vi "Enqueue Sync Await Release.vi"(8 "error in (no error)":errorcluster, 11 "Instrument Owner in":refnum<class "Instrument Owner.lvclass">) -> (0 "error out":errorcluster, 3 "Instrument Owner out":refnum<class "Instrument Owner.lvclass">)   [LabVIEW 2020, in "Instrument Handler.lvlib" / "Instrument Owner.lvclass"]
doc: "Await a notification on the Enqueue Sync notifier. Wait for Instrument Sequencer to complete the operation."
uses:
  Instrument Owner.lvclass
  Instrument Owner.lvclass/Instrument Owner.ctl
  PPL/HDH.Data.Generic.lvlibp/Synchronization/Notifier/Notifier.lvclass
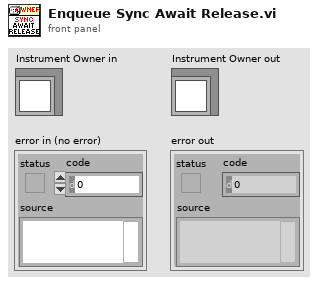
[diagram p1: front panel]
types:
  T1 = typedef "Instrument Handler.lvlib/Ctl_InstrumentSynchronicationCluster.ctl" = cluster{"Launched?":bool, "Driver Path":path, "Alias":string, "Connection Type":T2, "Pre Initialization Data":variant, "Enqueue Sync":refnum<class "Notifier.lvclass">, "Enqueue Lock":T3, "Owner Enqueuer":refnum<class "Message Enqueuer.lvclass">, "Owner":refnum<class "Sequencer Core.lvclass">, "Instrument ID":u32}
  T2 = typedef "HDH.Actor Framework.Core.Instrument Driver.lvlibp/Instrument Driver.lvclass/Ctl_ConnectionType.ctl" = enum16{"BuiltIn/System", "PXI/PCI", "USB", "GPIB", "VXI", "Serial", "TCP/IP", "cRIO", "SCXI", "cDAQ", "SwitchBlock", "SCC", "FireWire", "Accessory", "CAN", "SwitchBlock Device"}
  T3 = typedef "Semaphore RefNum" = refnum<k1>
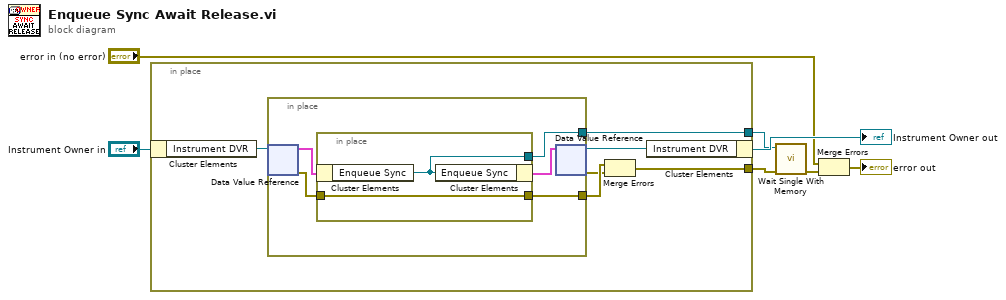
[diagram p0: block diagram]
diagram:
  n1 = in-place {
    in-place-border: [w10] -> w2
    in-place-border: [w8] -> w3
    n2 = in-place-cluster #1("Instrument Owner in") -> ("Instrument DVR"=w12:refnum<data-value>)
    n3 = in-place {
      in-place-border: [w18] -> w13
      in-place-border: [w14] -> w8
      n4 = in-place-dvr #2(w12) -> (w17:T1, w15:errorcluster)
      n5 = in-place {
        in-place-border: [w20] -> w18
        in-place-border: w15 -> [w20]
        in-place-border: [w19] -> w14
        n6 = in-place-cluster #3(w17) -> ("Enqueue Sync"=w19:refnum<class "Notifier.lvclass">)
        n7 = in-place-cluster #3("Enqueue Sync"=w19) -> (w16:T1)
      }
      n8 = in-place-dvr #2(w16) -> (w11:refnum<data-value>, w9:errorcluster)
    }
    n9 = Merge Errors(w13, w9) -> (w10:errorcluster)
    n10 = in-place-cluster #1("Instrument DVR"=w11) -> (→"Instrument Owner out":refnum<class "Instrument Owner.lvclass">)
  }
  n11 = call "Wait Single With Memory.vi"("error in (no error)"=w2, "Notifier in"=w3) -> ("error out"=w1:errorcluster)  [unwired: 6 in, 3 out]
  n12 = Merge Errors("error in (no error)", w1) -> (→"error out":errorcluster)
